vi "Convert_U16Img_to_Str_2.vi"(2 "error IN":errorcluster, 3 "[IN] U16 Pixel Img":u16[][](array[numeric])) -> (0 "error OUT":errorcluster, 1 "[OUT] Raw string":string)   [LabVIEW 2020]
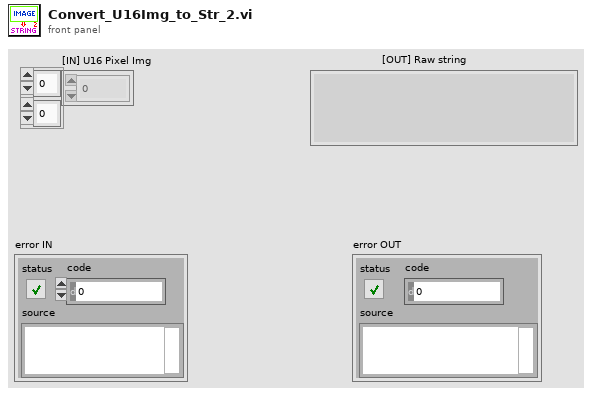
[diagram p1: front panel]
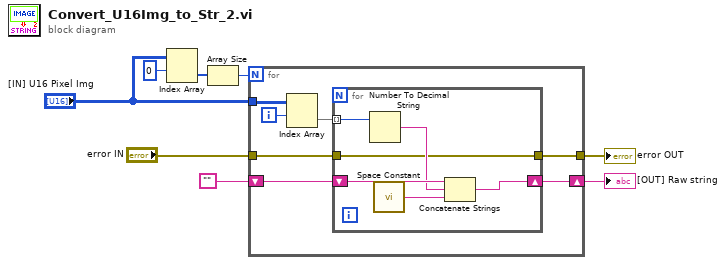
[diagram p0: block diagram]
diagram:
  n1 = Index Array(array="[IN] U16 Pixel Img", index (row)=0) -> (element=w7:u16[])  [unwired: 1 in]
  n2 = Array Size(array=w7) -> (size(s)=w6:i32)
  n3 = for {
    N: w6 -> [_]
    tunnel: "[IN] U16 Pixel Img" -> [w15]
    shift-right: [w11] -> w3
    shift-left: "" -> [w12]
    tunnel: "error IN" -> [w10]
    tunnel: [w9] -> w1
    i -> [w14]
    n4 = Index Array(array=w15, index (row)=w14) -> (element=w13:u16[])  [unwired: 1 in]
    n5 = for {
      tunnel: w13 -> [w21] mode=indexing
      shift-right: [w17] -> w11
      shift-left: w12 -> [w20]
      tunnel: w10 -> [w16]
      tunnel: [w16] -> w9
      n6 = Number To Decimal String(number=w21) -> (decimal integer string=w19:string)  [unwired: 1 in]
      n7 = call <vilib>:"Space Constant.vi"() -> ("String"=w18:string)
      n8 = Concatenate Strings(w20, w19, w18) -> (w17:string)
    }
  }
  "error OUT" <- w1
  "[OUT] Raw string" <- w3
